vi "Download_LatexPackages_Main.vi"   [LabVIEW 2014]
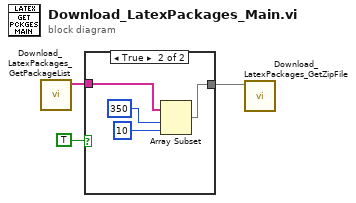
[diagram p0: block diagram]
diagram:
  n1 = call "Download_LatexPackages_GetPackageList.vi"() -> ("Array 2"=w3:string[])  [unwired: 11 in]
  n2 = case shown="True" TRUE {
    tunnel: w3 -> [w4 w8]
    tunnel: [w4 w7] -> w2
    frame False {
    }
    frame True {
      n3 = Array Subset(array=w8, index=350, length=10) -> (w7:string[])
    }
  }
  n4 = call "Download_LatexPackages_GetZipFile.vi"("package list (In)"=w2) -> ()  [unwired: 11 in]
